vi "3D-SubItem.vi"(10 "Col":i32, 11 "Pic Param  Data Collect":string[][](table)=[["", "", ""], ["", "", ""]]) -> (3 "ROI Output":T1 {"Rotation" format="%.2f"; "Left" scale=0.0..1024.0; "Right" scale=0.0..1024.0})   [LabVIEW 2011]
panel:
  in  "Rectangle":T1 {"Rotation" format="%.2f"; "Left" scale=0.0..1024.0; "Right" scale=0.0..1024.0}
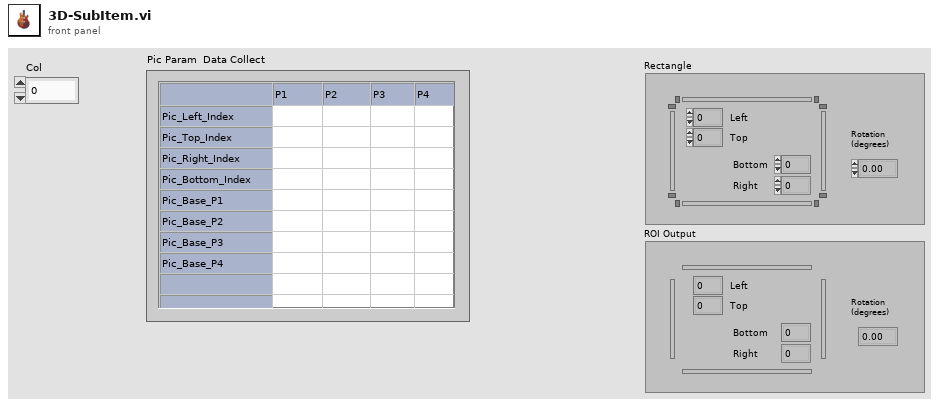
[diagram p1: front panel]
types:
  T1 = typedef "IMAQ Rectangle" = cluster{"Left":i32, "Top":i32, "Right":i32, "Bottom":i32, "Rotation":dbl}
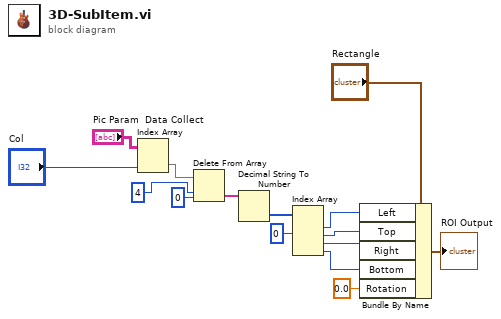
[diagram p0: block diagram]
diagram:
  n1 = Index Array(array="Pic Param  Data Collect", index (col)="Col") -> (element=w13:string[])  [unwired: 1 in]
  n2 = Delete From Array(array=w13, length=4 ("长度"), index=0 ("索引")) -> (deleted portion=w10:string[])  [unwired: 1 out]
  n3 = Decimal String To Number(string=w10) -> (number=w8:i32[])  [unwired: 2 in, 1 out]
  n4 = Index Array(array=w8, index #1=0 ("索引")) -> (element #1=w6:i32, element #2=w5:i32, element #3=w4:i32, element #4=w3:i32)  [unwired: 3 in]
  n5 = Bundle By Name(cluster="Rectangle", "Left"=w6, "Top"=w5, "Right"=w4, "Bottom"=w3, "Rotation"=0.0) -> (→"ROI Output":T1)
